vi "Make Texture.vi"(8 "Error In":errorcluster, 10 "Texture Name":string, 11 "WAD Cluster IN":T1) -> (0 "Error Out":errorcluster, 2 "2D Picture":picture, 3 "WAD Cluster OUT":T1)   [LabVIEW 2017]
uses:
  WAD_MainCluster.ctl
  TextureList.ctl
  PatchList.ctl
  Lumps.ctl
  <vilib>/picture/picture.llb/Draw 8-Bit Pixmap.vi
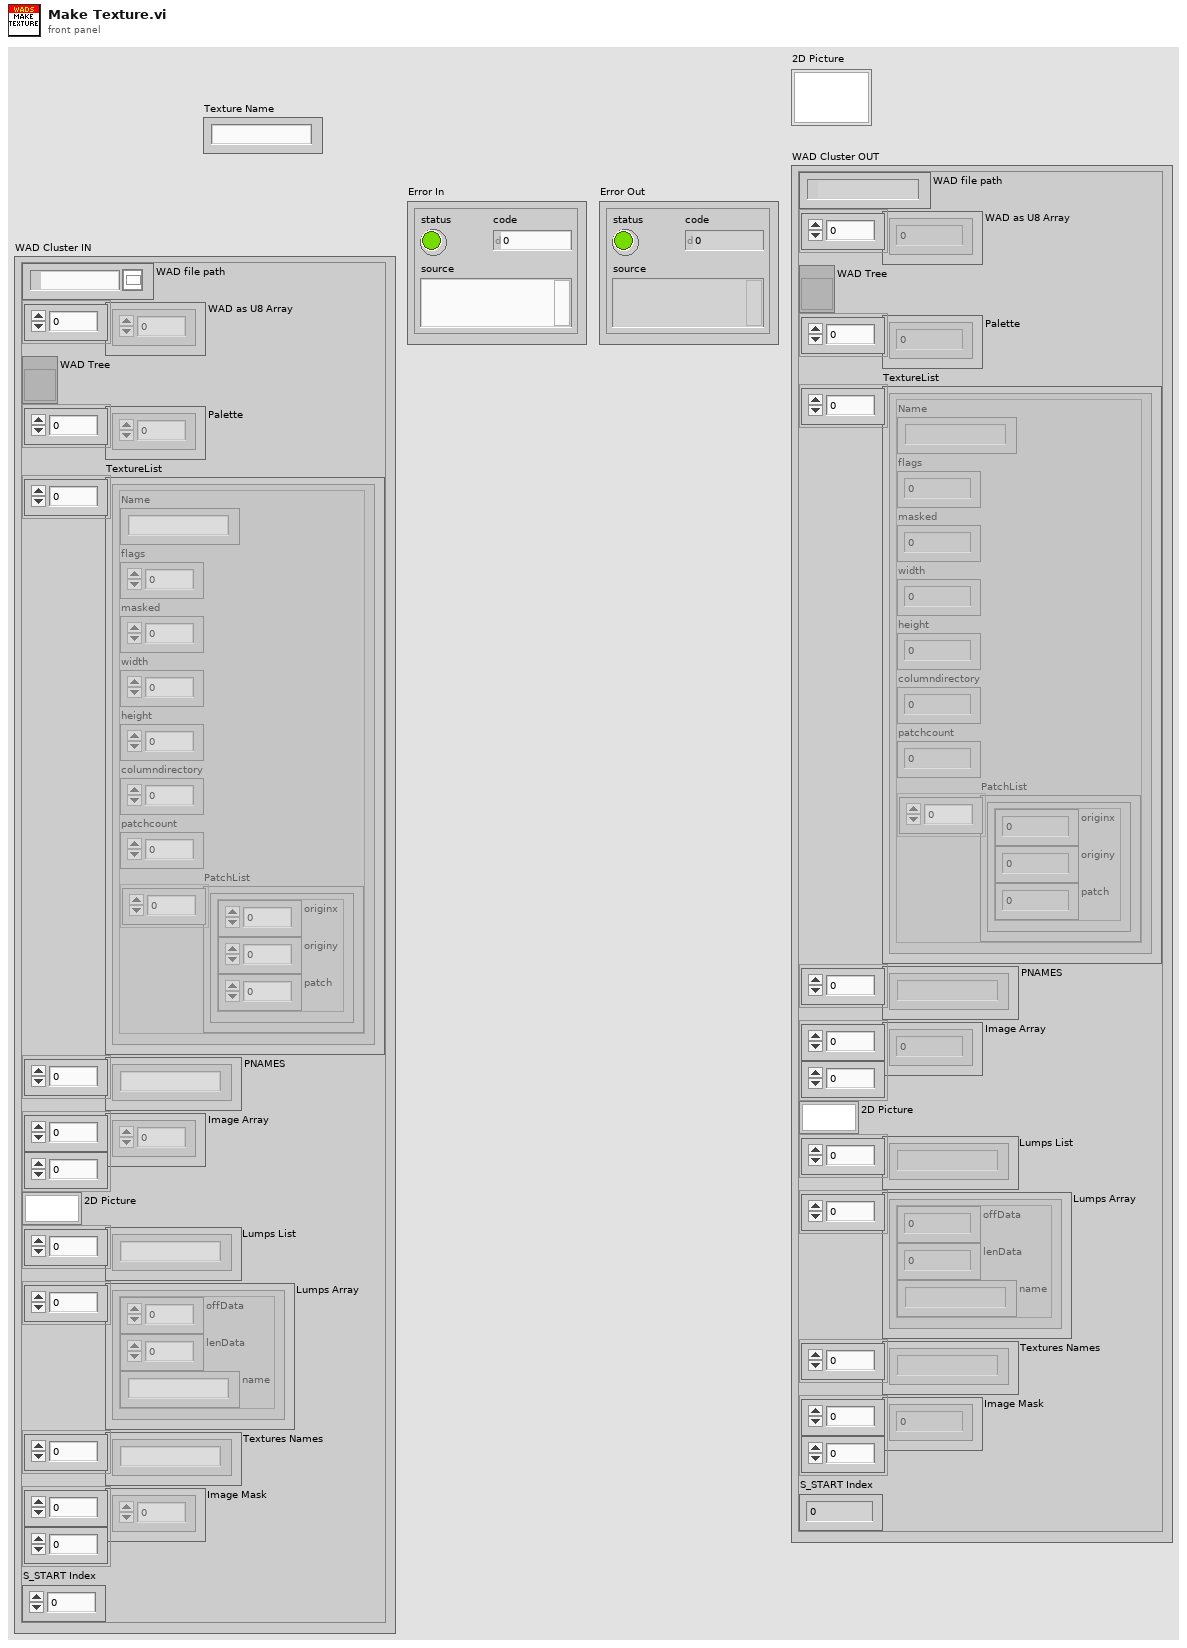
[diagram p1: front panel]
types:
  T1 = typedef "WAD_MainCluster.ctl" = cluster{"WAD file path":path, "WAD as U8 Array":u8[], "WAD Tree":refnum<vi>, "Palette":u32[], "TextureList":T2[], "PNAMES":string[], "Image Array":i16[][], "2D Picture":picture, "Lumps List":string[], "Lumps Array":T4[], "Textures Names":string[], "Image Mask":i16[][], "S_START Index":i32}
  T2 = typedef "TextureList.ctl" = cluster{"Name":string, "flags":u16, "masked":i16, "width":i16, "height":i16, "columndirectory":u32, "patchcount":i16, "PatchList":T3[]}
  T3 = typedef "PatchList.ctl" = cluster{"originx":i16, "originy":i16, "patch":i16}
  T4 = typedef "Lumps.ctl" = cluster{"offData":i32, "lenData":i32, "name":string}
  T5 = cluster{"left":i16, "top":i16, "right":i16, "bottom":i16}
  T6 = typedef "PatchHeader.ctl" = cluster{"Width":u16, "Height":u16, "XOffset":i16, "YOffset":i16}
  T7 = typedef "imagedata.ctl" = cluster{"image type":i32, "image depth":i32, "image":u8[], "mask":u8[], "colors":u32[], "Rectangle":cluster{"left":i16, "top":i16, "right":i16, "bottom":i16}}
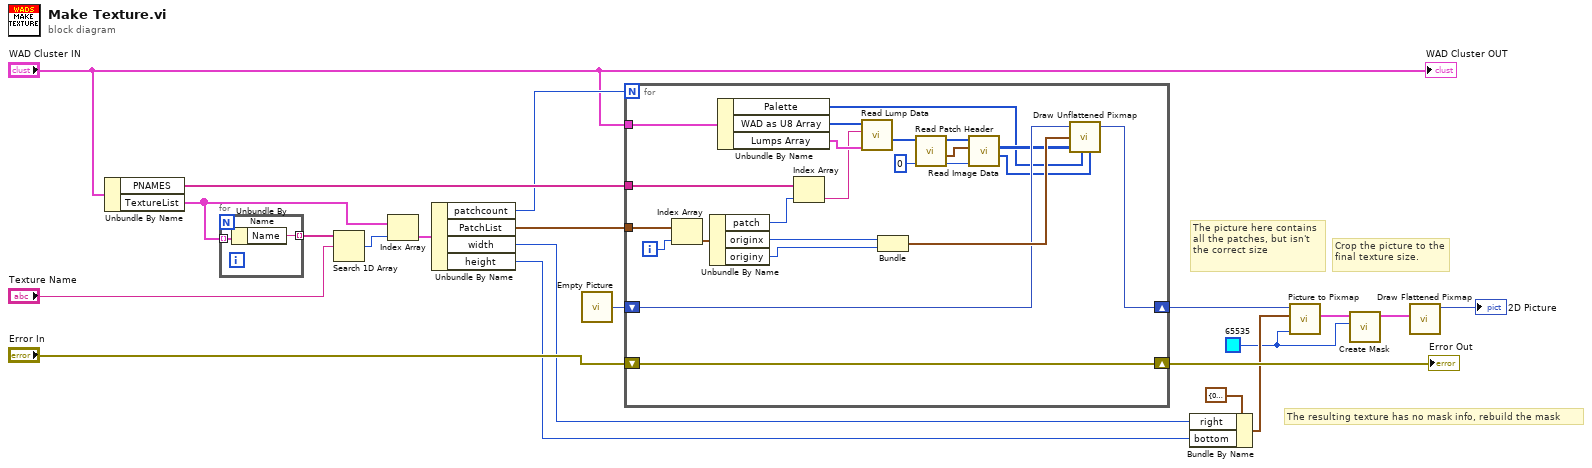
[diagram p0: block diagram]
diagram:
  w4 = u32 65535 ("Background Color")
  # "The resulting texture has no mask info, rebuild the mask"
  # "Crop the picture to the final texture size."
  # "The picture here contains all the patches, but isn't the correct size"
  n1 = Unbundle By Name("WAD Cluster IN") -> ("PNAMES"=w18:string[], "TextureList"=w14:T2[])
  n2 = for {
    tunnel: w14 -> [w23] mode=indexing
    tunnel: [w22] -> w13 mode=indexing
    n3 = Unbundle By Name(w23) -> ("Name"=w22:string)
  }
  n4 = Search 1D Array(1D array=w13, element="Texture Name") -> (index of element=w21:i32)  [unwired: 1 in]
  n5 = Index Array(array=w14, index=w21) -> (element=w19:T2)
  n6 = Unbundle By Name(w19) -> ("patchcount"=w17:i16, "PatchList"=w16:T3[], "width"=w9:i16, "height"=w8:i16)
  n7 = call "Empty Picture"() -> ("empty picture"=w1:picture)
  n8 = for {
    N: w17 -> [_]
    tunnel: w16 -> [w37]
    tunnel: w18 -> [w46]
    tunnel: "WAD Cluster IN" -> [w45]
    shift-right: [w27] -> w5
    shift-left: w1 -> [w31]
    shift-right: [w26] -> w15
    shift-left: "Error In" -> [w26]
    i -> [w36]
    n9 = Index Array(array=w37, index=w36) -> (element=w35:T3)
    n10 = Unbundle By Name(w35) -> ("patch"=w34:i16, "originx"=w25:i16, "originy"=w24:i16)
    n11 = Unbundle By Name(w45) -> ("Palette"=w28:u32[], "WAD as U8 Array"=w44:u8[], "Lumps Array"=w43:T4[])
    n12 = Index Array(array=w46, index=w34) -> (element=w33:string)
    n13 = call "Read Lump Data.vi"("Lumps Directory IN"=w43, "Lump Name"=w33, "Input U8"=w44) -> ("Lump DATA OUT"=w42:u8[])  [unwired: 5 in, 3 out]
    n14 = Bundle("originx"=w25, "originy"=w24) -> (w32:cluster{"originx":i16, "originy":i16})  [unwired: 1 in]
    n15 = call "Read Patch Header.vi"("Index"=u32 0, "Patch DATA IN"=w42) -> ("Index+8"=w38:u32, "PatchHeader"=w40:T6, "Patch DATA OUT"=w41:u8[])  [unwired: 7 in]
    n16 = call "Read Image Data.vi"("Input Index"=w38, "PatchHeader"=w40, "Patch DATA IN"=w41) -> ("Mask OUT"=w29:u8[], "Image OUT"=w30:u8[][])  [unwired: 5 in, 2 out]
    n17 = call-poly <vilib>:"Draw Unflattened Pixmap.vi"("picture"=w31, "top left point(0, 0)"=w32, "data"=w30, "color table"=w28, "mask"=w29) -> ("new picture"=w27:picture)  [unwired: 4 in]
  }
  "Error Out" <- w15
  n18 = Bundle By Name(cluster=T5 {"left"=0, "top"=0, "right"=0, "bottom"=0} ("rect"), "right"=w9, "bottom"=w8) -> (w7:T5)
  n19 = call <vilib>:"Picture to Pixmap.vi"("Background Color"=w4, "rect"=w7, "picture"=w5) -> ("image data"=w3:T7)  [unwired: 7 in, 1 out]
  n20 = call <vilib>:"Create Mask.vi"("Mask Color (Black)"=w4, "image data"=w3) -> ("image data"=w2:T7)  [unwired: 9 in]
  n21 = call <vilib>:"Draw Flattened Pixmap.vi"("image data"=w2) -> ("new picture"=→"2D Picture":picture)  [unwired: 8 in]
  "WAD Cluster OUT" <- "WAD Cluster IN"
